vi "Create AP Sx Object.vi"(6 "asicHandle":i32, 7 "asicName":string, 8 "error in (no error)":errorcluster caption="错误输入（无错误）", 9 "pgiChannel":i32, 10 "pgiDevNum":i32, 11 "pgiType":i32) -> (0 "error out":errorcluster caption="错误输出", 3 "function return":i32, 4 "asicHandle out":i32, 5 "asicName out":string)   [LabVIEW 2020]
doc: "extern int __stdcall CreateAPSxObject ( IN int pgiType, IN int pgiDevNum, IN int pgiChannel, IN char * asicName, OUT int * asicHandle);"
uses:
  APSx.dll/APSx.dll
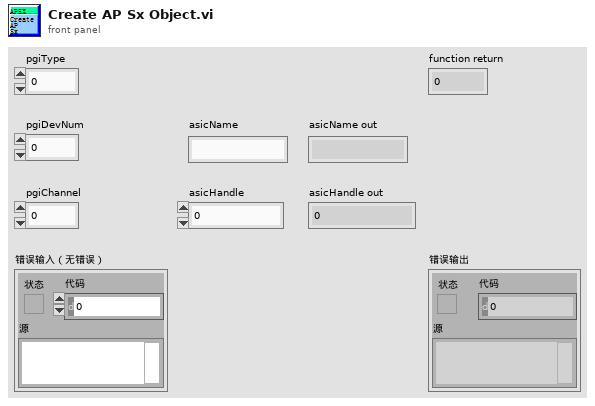
[diagram p1: front panel]
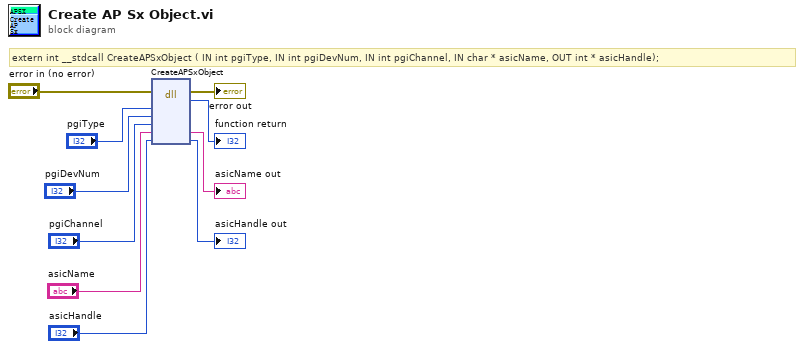
[diagram p0: block diagram]
diagram:
  # "extern int __stdcall CreateAPSxObject ( IN int pgiType, IN int pgiDevNum, IN int pgiChannel, IN char * asicName, OUT int * asicHandle);"
  n1 = dll-call lib="PTH2iabs CUsersFengDesktop传感器对中台传感器对中台labviewSourcesAPSx.dllAPSx.dll" fn="CreateAPSxObject"(error in="error in (no error)", "pgiType"="pgiType", "pgiDevNum"="pgiDevNum", "pgiChannel"="pgiChannel", "asicName"="asicName", "asicHandle"="asicHandle") -> (error out=→"error out":errorcluster, "返回类型"=→"function return":i32, "asicName"=→"asicName out":string, "asicHandle"=→"asicHandle out":i32)  [unwired: 5 in, 1 out]
